vi "Load_Store Sweep List.vi"(0 "VISA Resource Name":refnum<visa-resource-name>, 5 "Action (T:LOAD)":bool=TRUE, 9 "File Name (USER_SWEEP)":string="USER_SWEEP", 11 "error in (no error)":errorcluster {"code" format="%.0x"}) -> (4 "VISA Resource Name Out":refnum<visa-resource-name>, 15 "error out":errorcluster {"code" format="%.0x"})   [LabVIEW 2012, in "Agilent ESG Series.lvlib"]
doc: "This VI is used to load or store a sweep list from or to the specified file."
uses:
  <instrlib>/Agilent ESG Series/Agilent ESG Series.lvlib
panel:
  # "LOAD"
  # "STORE"
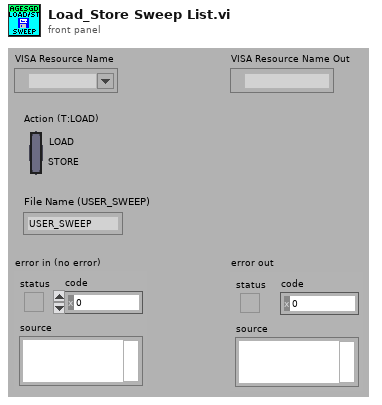
[diagram p1: front panel]
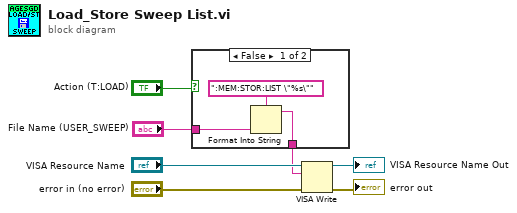
[diagram p0: block diagram]
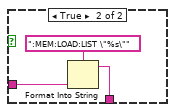
[diagram p2: hidden frame]
diagram:
  n1 = case shown="False" "Action (T:LOAD)" {
    tunnel: "File Name (USER_SWEEP)" -> [w9 w12]
    tunnel: [w8 w11] -> w5
    frame False {
      n2 = Format Into String(format string=":MEM:STOR:LIST \"%s\"", w9) -> (resulting string=w8:string)  [unwired: 2 in, 1 out]
    }
    frame True {
      n3 = Format Into String(format string=":MEM:LOAD:LIST \"%s\"", w12) -> (resulting string=w11:string)  [unwired: 2 in, 1 out]
    }
  }
  n4 = VISA Write(VISA resource name="VISA Resource Name", write buffer=w5, error in (no error)="error in (no error)") -> (VISA resource name out=→"VISA Resource Name Out":refnum<visa-resource-name>, error out=→"error out":errorcluster)  [unwired: 1 out]
